vi "Next Approved Submission.vi"(8 "error in (no error)":errorcluster, 11 "Submission DB in":refnum<class "Submission DB.lvclass">) -> (0 "error out":errorcluster, 1 "Found?":bool, 2 "Submission":refnum<class "Submission.lvclass">, 3 "Submission DB out":refnum<class "Submission DB.lvclass">)   [LabVIEW 2020, in "Summer of LabVIEW.lvlib" / "Submission DB.lvclass"]
uses:
  Submission DB.lvclass
  Submission/Submission.lvclass
  Submission DB.lvclass/Submission DB.ctl
  <vilib>/drjdpowell/SQLite Library/SQL Statement/SQL Statement.lvclass/SQL Statement.ctl
  <vilib>/drjdpowell/SQLite Library/SQL Statement/Step.vi
  <vilib>/drjdpowell/SQLite Library/SQL Statement/Error Message.vi
  SQLite/SQLite.lvclass
  <vilib>/drjdpowell/SQLite Library/SQL Connection/Connection.lvclass
  <vilib>/drjdpowell/SQLite Library/SQL Statement/SQL Statement.lvclass
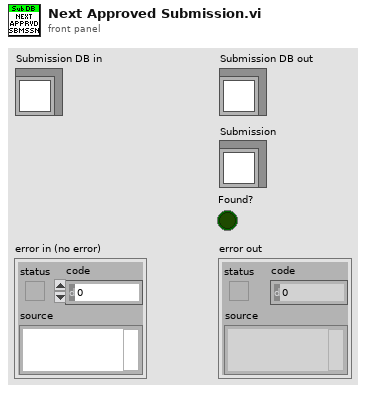
[diagram p1: front panel]
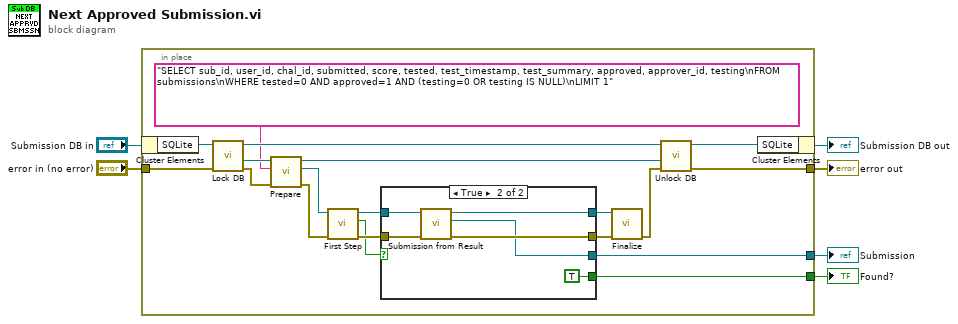
[diagram p0: block diagram]
diagram:
  n1 = in-place {
    in-place-border: "error in (no error)" -> [w24]
    in-place-border: [w21] -> w3
    in-place-border: [w12] -> w2
    in-place-border: [w7] -> w1
    n2 = in-place-cluster #1("Submission DB in") -> ("SQLite"=w25:refnum<class "SQLite.lvclass">)
    n3 = call "Lock DB.vi"("error in (no error)"=w24, "SQLite in"=w25) -> ("error out"=w17:errorcluster, "SQLite DB"=w20:refnum<class "Connection.lvclass">, "SQLite out"=w23:refnum<class "SQLite.lvclass">)  [unwired: 6 in, 1 out]
    n4 = call <vilib>:"Prepare.vi"("error in (no error)"=w17, "SQL"="SELECT sub_id, user_id, chal_id, submitted, score, tested, test_timestamp, test_summary, approved, approver_id, testing\nFROM submissions\nWHERE tested=0 AND approved=1 AND (testing=0 OR testing IS NULL)\nLIMIT 1", "SQLite Connection in"=w20) -> ("error out"=w16:errorcluster, "SQL Statement"=w18:refnum<class "SQL Statement.lvclass">, "SQLite Connection"=w8:refnum<class "Connection.lvclass">)  [unwired: 4 in, 2 out]
    n5 = call <vilib>:"First Step.vi"("error in (no error)"=w16, "SQL Statement in"=w18) -> ("error out"=w15:errorcluster, "Row returned"=w14:bool, "SQL Statement"=w13:refnum<class "SQL Statement.lvclass">)  [unwired: 7 in]
    n6 = case shown="True" w14 {
      tunnel: w15 -> [w26 w32]
      tunnel: w13 -> [w27 w33]
      tunnel: [w27 w31] -> w11
      tunnel: [w26 w30] -> w10
      tunnel: [_ w29] -> w12
      tunnel: [_ TRUE] -> w7
      frame False {
      }
      frame True {
        n7 = call "Submission from Result.vi"("error in (no error)"=w32, "Statement In"=w33) -> ("error out"=w30:errorcluster, "Submission"=w29:refnum<class "Submission.lvclass">, "Statement"=w31:refnum<class "SQL Statement.lvclass">)  [unwired: 7 in]
      }
    }
    n8 = call <vilib>:"Finalize.vi"("error in (no error)"=w10, "SQL Statement in"=w11) -> ("error out"=w9:errorcluster)  [unwired: 9 in]
    n9 = call "Unlock DB.vi"("error in (no error)"=w9, "SQLite DB"=w8, "SQLite in"=w23) -> ("error out"=w21:errorcluster, "SQLite out"=w22:refnum<class "SQLite.lvclass">)  [unwired: 7 in]
    n10 = in-place-cluster #1("SQLite"=w22) -> (→"Submission DB out":refnum<class "Submission DB.lvclass">)
  }
  "error out" <- w3
  "Submission" <- w2
  "Found?" <- w1
